vi "CRCTest.vi"() -> ()   [LabVIEW 2018]
uses:
  <vilib>/rvi/Emulation/niFpgaSctlEmulationGetInTimedLoop.vi
  <vilib>/Utility/error.llb/Clear Errors.vi
  <vilib>/rvi/DataTransferAndStorage/Container/Common/niFpgaContainerGetUniqueNameForEmu.vi
  <vilib>/rvi/DataTransferAndStorage/Container/Common/niFpgaContainerSetEmuInfo.vi
  <vilib>/rvi/eio/common/nirviEmuReportErrorAndStop.vi
  <vilib>/rvi/DataTransferAndStorage/Container/Common/niFpgaContainerExecOnDevCompGetState.vi
  <vilib>/rvi/Emulation/niFpgaEmulationIsFPGAContextNoSignature.vi
  <vilib>/rvi/Emulation/niFpgaProcessEmulError.vi
  <vilib>/rvi/errors/nirviReportUnexpectedCaseInternalError (U32).vi
  <vilib>/rvi/Memory/Memory_Emulation/niFpgaMemoryEmulationCacheClearOnFirstRun.vi
  <vilib>/rvi/Memory/Memory_Emulation/nirvimemoryEmulationManagerCache_MakeExclusive.vi
  <vilib>/rvi/Memory/Memory_Emulation/niFpgaMemoryEmulationValidateCache.vi
  <vilib>/rvi/Memory/Memory_Emulation/nirvimemoryEmulationManagerCache_InsertValue.vi
  <vilib>/rvi/Memory/Memory_Emulation/nirvimemoryEmulationManagerCache_ReleaseExclusive.vi
  <vilib>/rvi/Memory/Memory_Emulation/nirvimemoryEmulationManagerCache_GetValue.vi
  <vilib>/rvi/Memory/Memory_Emulation/nirvimemoryEmulationManagerCache_SetValue.vi
  <vilib>/rvi/Emulation/niFpgaSctlEmulationResourceMgr.vi
  <vilib>/rvi/LocalResourceManager/LocalResourceManager.xnode
  <vilib>/rvi/DataTransferAndStorage/Container/XNode/niFpgaContainer.xnode
  <vilib>/rvi/Memory/Memory_Emulation/niFpgaMemoryEmulationRefIn.vi
  Modbus_Processing_Unit.lvlib
panel:
  in  "Offset":i16
  in  "Size":u8
  out "CRC Lo":u8
  out "CRC Hi":u8
  in  "Data":u8[](array[numeric])
  # "Calculates ModBus 16 bit CRC\n\nInput is array of uint8 values. Output is two\nuint8 values, representing CRC."
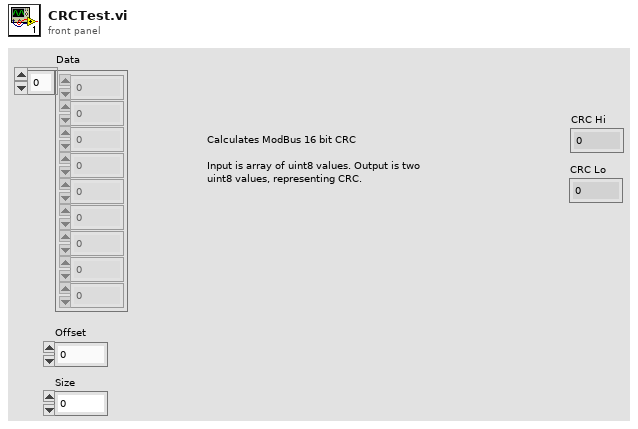
[diagram p1: front panel]
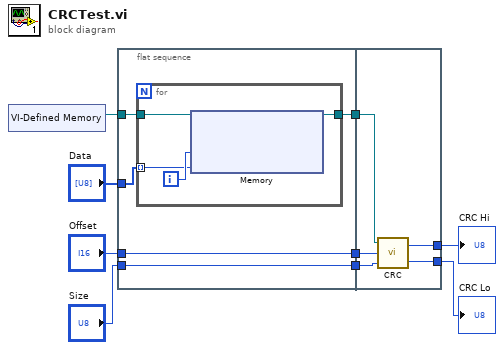
[diagram p0: block diagram]
diagram:
  n1 = xnode "VI-Defined Memory"() -> ("Memory Out"=w2:refnum<k21>)
  n2 = flat-sequence {
    tunnel: "Size" -> [w13]
    tunnel: "Offset" -> [w14]
    tunnel: [w14] -> w5
    tunnel: [w13] -> w4
    tunnel: "Data" -> [w11]
    tunnel: w2 -> [w12]
    tunnel: [w10] -> w1
    tunnel: [w21] -> w7
    tunnel: [w20] -> w6
    tunnel: w5 -> [w23]
    tunnel: w4 -> [w22]
    tunnel: w1 -> [w19]
    frame #0 {
      n3 = for {
        tunnel: w12 -> [w18]
        tunnel: w11 -> [w16] mode=indexing
        tunnel: [w15] -> w10
        i -> [w17]
        n4 = xnode "Memory"("Address"=w17, "Data"=w16, "Memory In"=w18) -> ("Memory Out"=w15:refnum<k21>)
      }
    }
    frame #1 {
      n5 = call "CRC.vi"("Size"=w22, "Offset"=w23, "Data"=w19) -> ("CRC Lo"=w21:u8, "CRC Hi"=w20:u8)
    }
  }
  "CRC Hi" <- w6
  "CRC Lo" <- w7
